vi "Str to Value.vi"(8 "error in":errorcluster, 10 "DefaultValue":string, 11 "DataType":T1=enum."U8") -> (0 "error out":errorcluster, 3 "Variant":variant)   [LabVIEW 2025, in "PLC_Module.lvlib" / "PLC_Module.lvclass"]
uses:
  PLC_Module.lvclass
  PLC_Data_Type.ctl
  158c854f-5f36-4f39-8c0c-1abd5f6353ad.vi
  04392f00-7449-4373-9e72-4409eebb5169.vi
  d22f31f2-30f0-4861-818d-67902c36ff5b.vi
  0fc07c9d-2ab0-41c8-9327-1a2c065f7ccf.vi
  <vilib>/JDP Science/JSONtext/JSON text to Variant.vi
  <vilib>/JDP Science/JSONtext/LVClass Serializer/JSONtext LVClass Serializer.lvclass
  PLC_Module.lvclass/PLC_Module.ctl
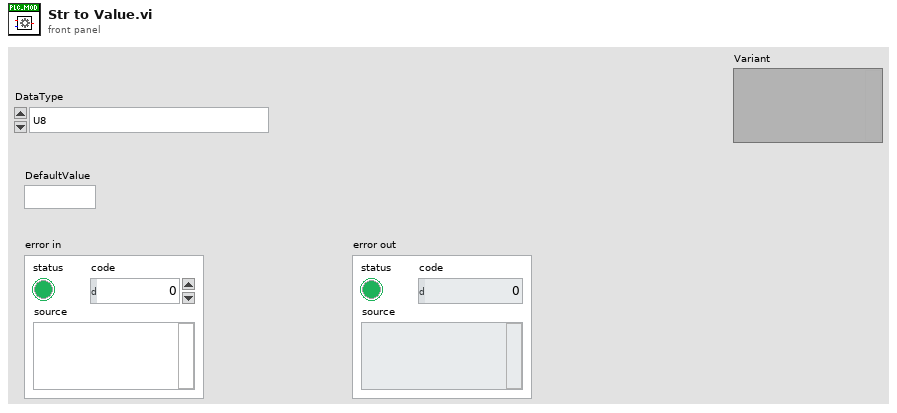
[diagram p1: front panel]
types:
  T1 = typedef "PLC_Module.lvlib/PLC_Module.lvclass/PLC_Data_Type.ctl" = enum16{"Boolean", "Single Float", "U8", "U32", "U32_Array", "String"}
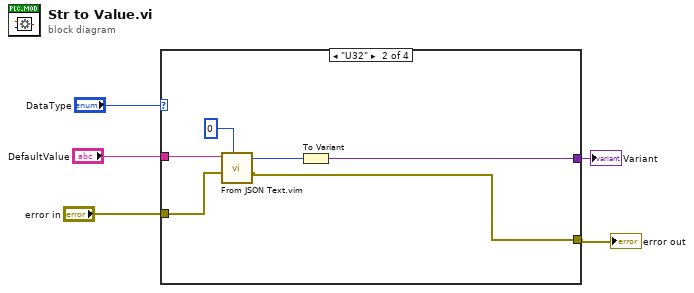
[diagram p0: block diagram]
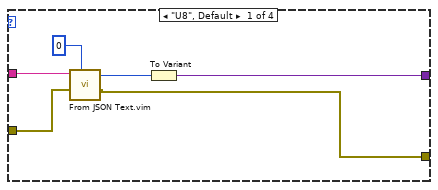
[diagram p2: hidden frame]
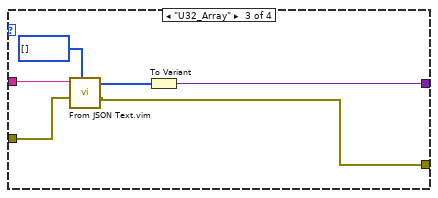
[diagram p3: hidden frame]
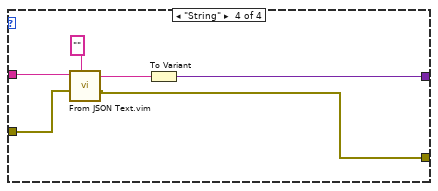
[diagram p4: hidden frame]
diagram:
  n1 = case shown="\"U32\"" "DataType" {
    tunnel: "DefaultValue" -> [w11 w17 w23 w29]
    tunnel: "error in" -> [w8 w14 w21 w27]
    tunnel: [w7 w13 w20 w26] -> w2
    tunnel: [w6 w12 w19 w25] -> w1
    frame "U8", Default {
      n2 = call "From JSON Text.vim"("Data Type and Default Value"=u8 0, "error in (no error)"=w8, "JSON"=w11) -> ("error out"=w7:errorcluster, "Data out"=w9:u8)  [unwired: 7 in]
      n3 = To Variant(anything=w9) -> (Variant=w6:variant)
    }
    frame "U32" {
      n4 = call "From JSON Text.vim"("Data Type and Default Value"=u32 0, "error in (no error)"=w14, "JSON"=w17) -> ("error out"=w13:errorcluster, "Data out"=w15:u32)  [unwired: 7 in]
      n5 = To Variant(anything=w15) -> (Variant=w12:variant)
    }
    frame "U32_Array" {
      n6 = call "From JSON Text.vim"("Data Type and Default Value"=u32[] [], "error in (no error)"=w21, "JSON"=w23) -> ("error out"=w20:errorcluster, "Data out"=w22:u32[])  [unwired: 7 in]
      n7 = To Variant(anything=w22) -> (Variant=w19:variant)
    }
    frame "String" {
      n8 = call "From JSON Text.vim"("Data Type and Default Value"="", "error in (no error)"=w27, "JSON"=w29) -> ("error out"=w26:errorcluster, "Data out"=w28:string)  [unwired: 7 in]
      n9 = To Variant(anything=w28) -> (Variant=w25:variant)
    }
  }
  "error out" <- w2
  "Variant" <- w1
